vi "2_LI_COR.vi"() -> ()   [LabVIEW 2013]
panel:
  out "Water Temperature":dbl(slide) scale=0.0..30.0
  out "?":dbl(slide) scale=0.0..1200.0
  out "?":dbl(slide) scale=0.0..1200.0
  out "Diffuse Irradiance (W/m^2)":dbl format="%#_4g"
  out "Direct Irradiance (W/m^2)":dbl format="%#_4g"
  out "Irradiance vs Time":dynamicdata(graph)
  in  "Stop VI":bool
  in  "Save Data":bool
  in  "File Location":path=path "\\\\EGRSHARES\\Homes/NAU-STUDENTS/el335/Documents/Labview Test/LVtest1.lvm" caption="Filename"
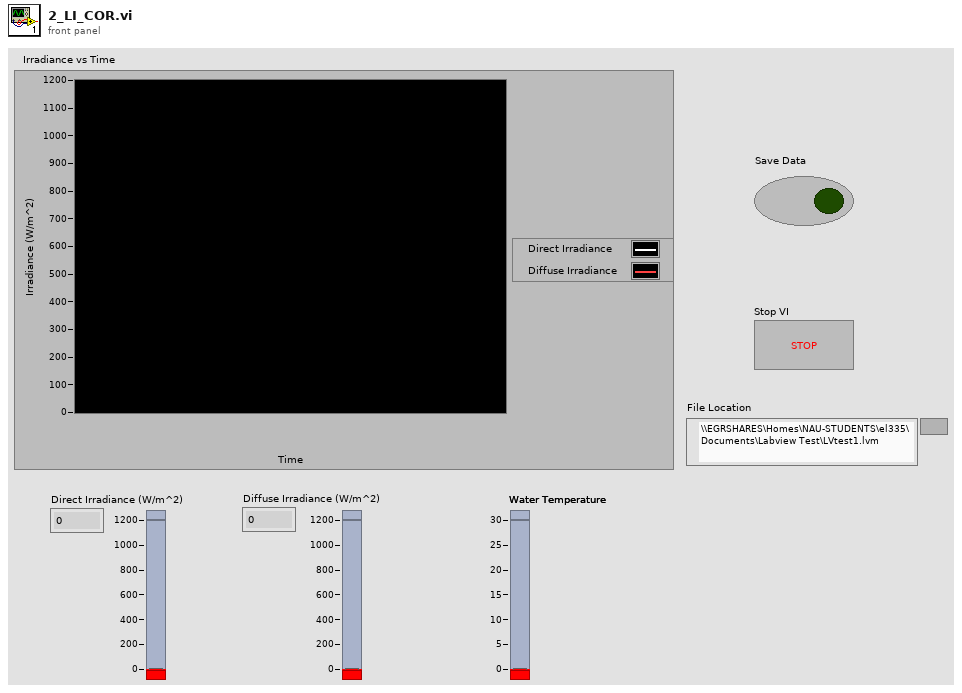
[diagram p1: front panel]
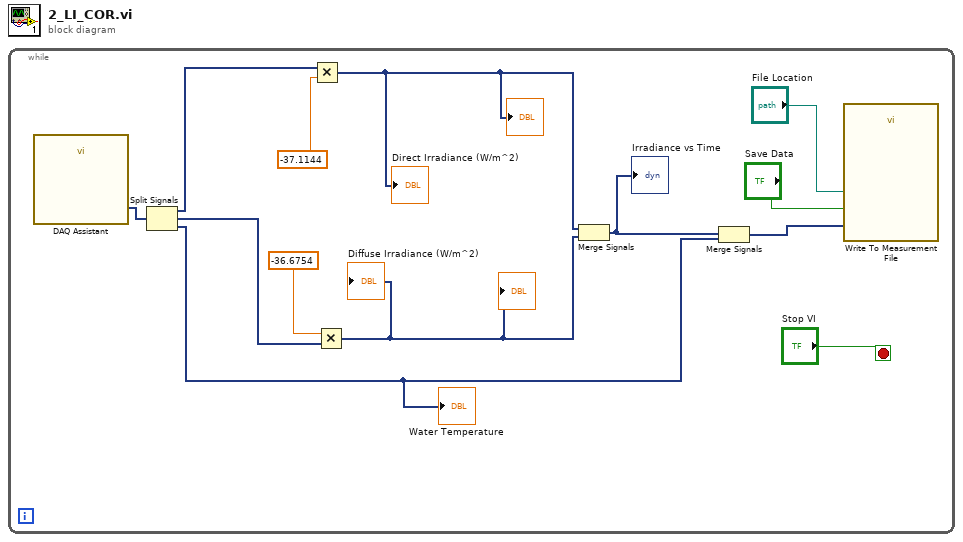
[diagram p0: block diagram]
diagram:
  n1 = while {
    stop <- "Stop VI" stop-if-true
    n2 = call "DAQ Assistant"() -> ("data"=w10:dynamicdata)  [unwired: 16 in, 3 out]
    n3 = Split Signals(w10) -> (w4:dynamicdata, w9:dynamicdata, w5:dynamicdata)  [unwired: 3 in]
    "Water Temperature" <- w5
    n4 = Multiply(x=w4, y=-37.1144) -> (x*y=w6:dynamicdata)
    "Direct Irradiance (W/m^2)" <- w6
    "?" <- w6
    n5 = Multiply(x=-36.6754, y=w9) -> (x*y=w3:dynamicdata)
    "Diffuse Irradiance (W/m^2)" <- w3
    "?" <- w3
    n6 = Merge Signals(w6, w3) -> (w7:dynamicdata)
    "Irradiance vs Time" <- w7
    n7 = Merge Signals(w7, w5) -> (w8:dynamicdata)
    n8 = call "Write To Measurement File"("Signals"=w8, "Enable"="Save Data", "Filename"="File Location") -> ()  [unwired: 14 in, 3 out]
  }
